vi "SelectAutoFile.vi"(8 "Routine":T1 items=["Definately Switch", "Definately Scale", "Switch if in front, else scale", "Scale if in front, else switch", "Switch if in front, else nothing", "Scale if in front, else nothing", "Drive across line"], 9 "OurSwitch":bool, 10 "OurScale":bool, 11 "Position":dbl) -> (3 "File Name":string)   [LabVIEW 2017]
uses:
  Shared/AutoRoutineSelector.ctl
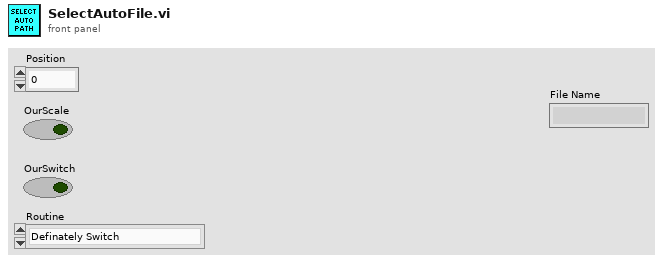
[diagram p1: front panel]
types:
  T1 = typedef "AutoRoutineSelector.ctl" = u16
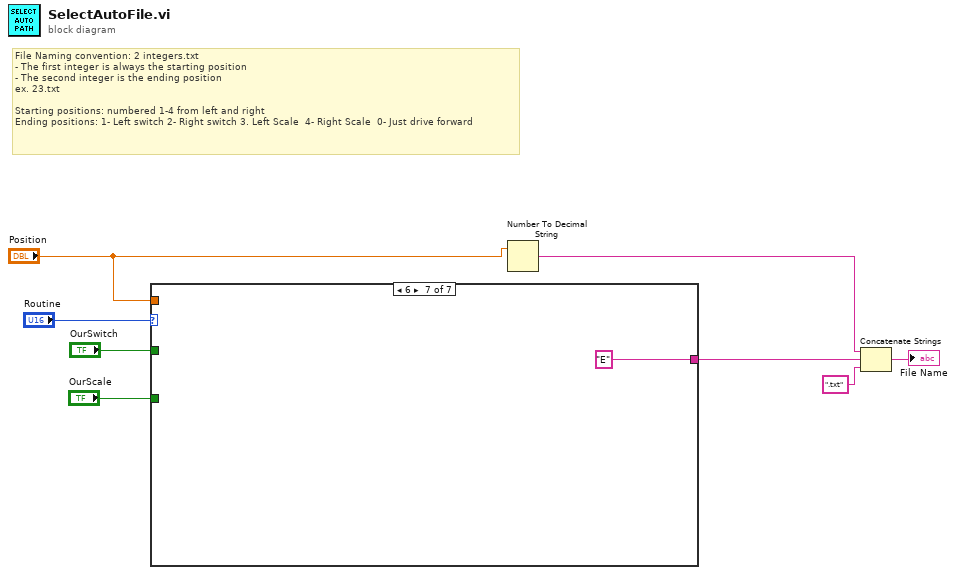
[diagram p0: block diagram]
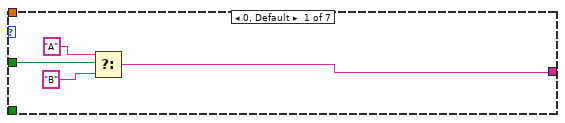
[diagram p2: hidden frame]
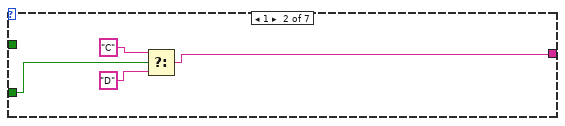
[diagram p3: hidden frame]
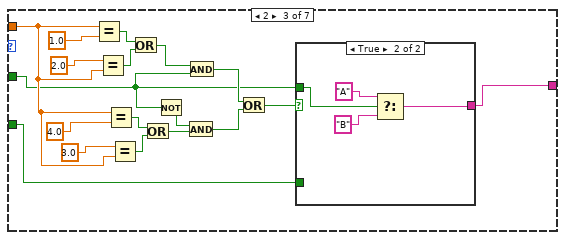
[diagram p4: hidden frame]
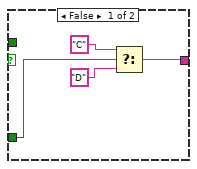
[diagram p5: hidden frame]
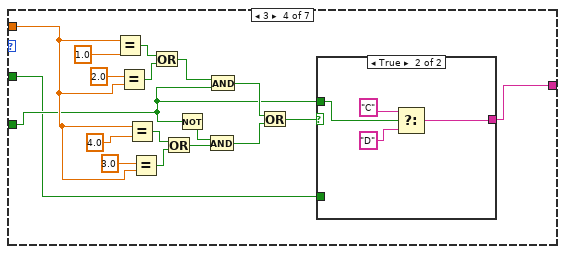
[diagram p6: hidden frame]
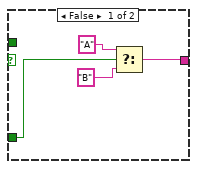
[diagram p7: hidden frame]
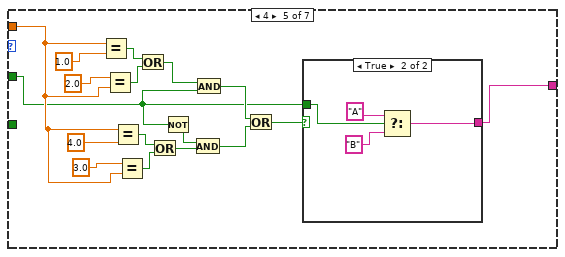
[diagram p8: hidden frame]
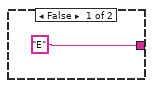
[diagram p9: hidden frame]
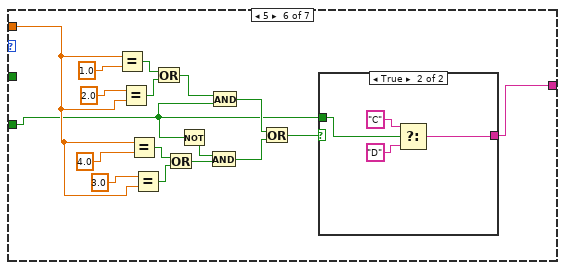
[diagram p10: hidden frame]
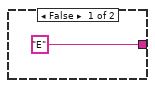
[diagram p11: hidden frame]
diagram:
  # "File Naming convention: 2 integers.txt \n- The first integer is always the starting position\n- The second integer is the ending position\nex. 23.txt\n\nStarting positions: numbered 1-4 from left and right\nEnding positions: 1- Left switch 2- Right switch 3. Left Scale  4- Right Scale  0- Just drive forward"
  n1 = case shown="6" "Routine" {
    tunnel: "OurSwitch" -> [w12 _ w23 w48 w74 _ _]
    tunnel: "OurScale" -> [_ w16 w22 w49 _ w96 _]
    tunnel: [w9 w13 w17 w43 w69 w91 "E"] -> w1
    tunnel: "Position" -> [_ _ w29 w50 w75 w97 _]
    frame 0, Default {
      n2 = Select(t="A", s=w12, f="B") -> (s? t:f=w9:string)
    }
    frame 1 {
      n3 = Select(t="C", s=w16, f="D") -> (s? t:f=w13:string)
    }
    frame 2 {
      n4 = Equal?(x=w29, y=1.0) -> (x = y?=w34:bool)
      n5 = Equal?(x=2.0 ("y"), y=w29) -> (x = y?=w33:bool)
      n6 = Equal?(x=w29, y=4.0) -> (x = y?=w30:bool)
      n7 = Equal?(x=3.0 ("y"), y=w29) -> (x = y?=w31:bool)
      n8 = Or(x=w34, y=w33) -> (x .or. y?=w32:bool)
      n9 = Or(x=w30, y=w31) -> (x .or. y?=w28:bool)
      n10 = Not(x=w23) -> (.not. x?=w27:bool)
      n11 = And(x=w27, y=w28) -> (x .and. y?=w25:bool)
      n12 = And(x=w32, y=w23) -> (x .and. y?=w26:bool)
      n13 = Or(x=w26, y=w25) -> (x .or. y?=w24:bool)
      n14 = case shown="True" w24 {
        tunnel: w23 -> [_ w42]
        tunnel: [w37 w39] -> w17
        tunnel: w22 -> [w38 _]
        frame False {
          n15 = Select(t="C", s=w38, f="D") -> (s? t:f=w37:string)
        }
        frame True {
          n16 = Select(t="A", s=w42, f="B") -> (s? t:f=w39:string)
        }
      }
    }
    frame 3 {
      n17 = Equal?(x=w50, y=1.0) -> (x = y?=w51:bool)
      n18 = Equal?(x=2.0 ("y"), y=w50) -> (x = y?=w52:bool)
      n19 = Equal?(x=w50, y=4.0) -> (x = y?=w55:bool)
      n20 = Equal?(x=3.0 ("y"), y=w50) -> (x = y?=w54:bool)
      n21 = Or(x=w51, y=w52) -> (x .or. y?=w53:bool)
      n22 = Or(x=w55, y=w54) -> (x .or. y?=w56:bool)
      n23 = Not(x=w49) -> (.not. x?=w57:bool)
      n24 = And(x=w57, y=w56) -> (x .and. y?=w59:bool)
      n25 = And(x=w53, y=w49) -> (x .and. y?=w58:bool)
      n26 = Or(x=w58, y=w59) -> (x .or. y?=w60:bool)
      n27 = case shown="True" w60 {
        tunnel: w49 -> [_ w68]
        tunnel: [w63 w65] -> w43
        tunnel: w48 -> [w64 _]
        frame False {
          n28 = Select(t="A", s=w64, f="B") -> (s? t:f=w63:string)
        }
        frame True {
          n29 = Select(t="C", s=w68, f="D") -> (s? t:f=w65:string)
        }
      }
    }
    frame 4 {
      n30 = Equal?(x=w75, y=1.0) -> (x = y?=w76:bool)
      n31 = Equal?(x=2.0 ("y"), y=w75) -> (x = y?=w77:bool)
      n32 = Equal?(x=w75, y=4.0) -> (x = y?=w80:bool)
      n33 = Equal?(x=3.0 ("y"), y=w75) -> (x = y?=w79:bool)
      n34 = Or(x=w76, y=w77) -> (x .or. y?=w78:bool)
      n35 = Or(x=w80, y=w79) -> (x .or. y?=w81:bool)
      n36 = Not(x=w74) -> (.not. x?=w82:bool)
      n37 = And(x=w82, y=w81) -> (x .and. y?=w84:bool)
      n38 = And(x=w78, y=w74) -> (x .and. y?=w83:bool)
      n39 = Or(x=w83, y=w84) -> (x .or. y?=w85:bool)
      n40 = case shown="True" w85 {
        tunnel: w74 -> [_ w90]
        tunnel: ["E" w87] -> w69
        frame False {
        }
        frame True {
          n41 = Select(t="A", s=w90, f="B") -> (s? t:f=w87:string)
        }
      }
    }
    frame 5 {
      n42 = Equal?(x=w97, y=1.0) -> (x = y?=w107:bool)
      n43 = Equal?(x=2.0 ("y"), y=w97) -> (x = y?=w106:bool)
      n44 = Equal?(x=w97, y=4.0) -> (x = y?=w103:bool)
      n45 = Equal?(x=3.0 ("y"), y=w97) -> (x = y?=w104:bool)
      n46 = Or(x=w107, y=w106) -> (x .or. y?=w105:bool)
      n47 = Or(x=w103, y=w104) -> (x .or. y?=w102:bool)
      n48 = Not(x=w96) -> (.not. x?=w101:bool)
      n49 = And(x=w101, y=w102) -> (x .and. y?=w99:bool)
      n50 = And(x=w105, y=w96) -> (x .and. y?=w100:bool)
      n51 = Or(x=w100, y=w99) -> (x .or. y?=w98:bool)
      n52 = case shown="True" w98 {
        tunnel: w96 -> [_ w112]
        tunnel: ["E" w109] -> w91
        frame False {
        }
        frame True {
          n53 = Select(t="C", s=w112, f="D") -> (s? t:f=w109:string)
        }
      }
    }
    frame 6 {
    }
  }
  n54 = Number To Decimal String(number="Position") -> (decimal integer string=w6:string)  [unwired: 1 in]
  n55 = Concatenate Strings(w6, w1, ".txt") -> (→"File Name":string)
